vi "Initialize Tag.vi"(6 "Units":string, 8 "error in (no error)":errorcluster, 9 "Data Type":string(combo), 10 "Tag Path":string, 11 "Logger in.lvclass":refnum<class "Logger.lvclass">) -> (0 "error out":errorcluster, 3 "Logger out.lvclass":refnum<class "Logger.lvclass">)   [LabVIEW 2016, in "Logger.lvclass"]
uses:
  Logger.lvclass
  Logger.lvclass/Logger.ctl
  <vilib>/TagLibrary/Create Tag (String).vi
  <vilib>/TagLibrary/Create Tag (Int).vi
  <vilib>/TagLibrary/Create Tag (Double).vi
  <vilib>/TagLibrary/TagLibrary.lvlib
  <resource>/objmgr/niTag.rc
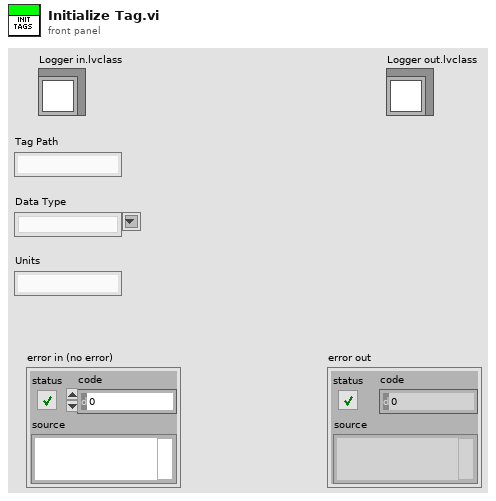
[diagram p1: front panel]
types:
  T1 = cluster{"Tag Reference":refnum<k21>, "Tag Units":string, "Tag Path":string, "Waveform":waveform(dbl), "Log":bool}
  T2 = cluster{"Tag Reference":refnum<k21>, "Tag Units":string, "Tag Path":string, "Waveform":waveform(dbl), "Log":bool}[]
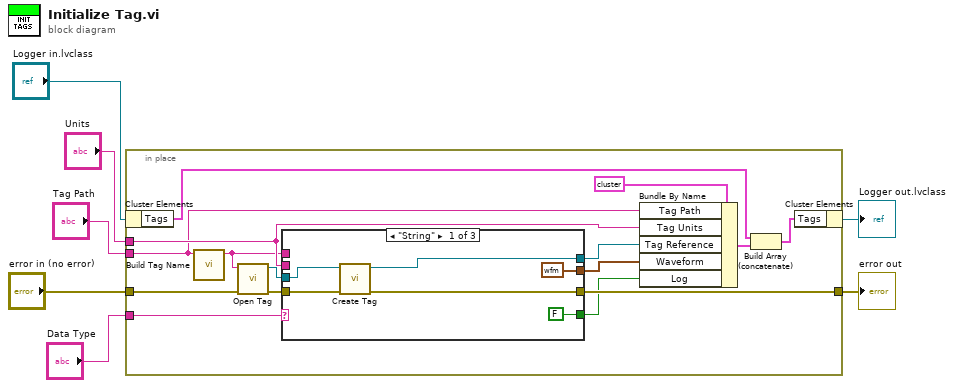
[diagram p0: block diagram]
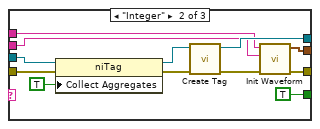
[diagram p2: hidden frame]
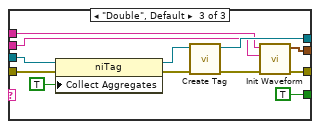
[diagram p3: hidden frame]
diagram:
  n1 = in-place {
    in-place-border: [w20] -> w7
    in-place-border: "Tag Path" -> [w8]
    in-place-border: "Data Type" -> [w19]
    in-place-border: "Units" -> [w16]
    in-place-border: "error in (no error)" -> [w15]
    n2 = in-place-cluster #1("Logger in.lvclass") -> ("Tags"=w11:T2)
    n3 = call "Build Tag Name.vi"("Tag"=w8) -> ("System Tag"=w12:string)  [unwired: 9 in, 1 out]
    n4 = call <vilib>:"Open Tag.vi"("error in (no error)"=w15, "tag path"=w12) -> ("error out"=w21:errorcluster, "tag reference out"=w22:refnum<k21>)  [unwired: 8 in]
    n5 = case shown="\"String\"" w19 {
      tunnel: w22 -> [w28 w40 w52]
      tunnel: w21 -> [w27 w37 w49]
      tunnel: [w25 w32 w44] -> w20
      tunnel: [w26 w35 w47] -> w17
      tunnel: [FALSE TRUE TRUE] -> w13
      tunnel: w16 -> [_ w29 w41]
      tunnel: [waveform(dbl) {"t0"=timestamp(0 s since 1904-01-01), "dt"=1.0, "Y"=[]} ("waveform") w31 w43] -> w14
      tunnel: w12 -> [_ w30 w42]
      frame "String" {
        n6 = call-poly <vilib>:"Create Tag.vi"("error in (no error)"=w27, "tag reference in"=w28) -> ("error out"=w25:errorcluster, "tag reference out"=w26:refnum<k21>)  [unwired: 8 in]
      }
      frame "Integer" {
        n7 = property class="niTag"(reference=w40, error in=w37, "Collect Aggregates"=TRUE) -> (reference out=w39:refnum<k21>, error out=w38:errorcluster)
        n8 = call-poly <vilib>:"Create Tag.vi"("error in (no error)"=w38, "tag reference in"=w39) -> ("error out"=w33:errorcluster, "tag reference out"=w35:refnum<k21>)  [unwired: 8 in]
        n9 = call "Init Waveform.vi"("error in (no error)"=w33, "Units"=w29, "System Tag"=w30) -> ("error out"=w32:errorcluster, "waveform"=w31:waveform(dbl))  [unwired: 7 in]
      }
      frame "Double", Default {
        n10 = property class="niTag"(reference=w52, error in=w49, "Collect Aggregates"=TRUE) -> (reference out=w51:refnum<k21>, error out=w50:errorcluster)
        n11 = call-poly <vilib>:"Create Tag.vi"("error in (no error)"=w50, "tag reference in"=w51) -> ("error out"=w45:errorcluster, "tag reference out"=w47:refnum<k21>)  [unwired: 8 in]
        n12 = call "Init Waveform.vi"("error in (no error)"=w45, "Units"=w41, "System Tag"=w42) -> ("error out"=w44:errorcluster, "waveform"=w43:waveform(dbl))  [unwired: 7 in]
      }
    }
    n13 = Bundle By Name(cluster=T1 {"Tag Reference"="", "Tag Units"="", "Tag Path"="", "Waveform"={"t0"=timestamp(0 s since 1904-01-01), "dt"=1.0, "Y"=[]}, "Log"=FALSE} ("Tag"), "Tag Path"=w8, "Tag Units"=w16, "Tag Reference"=w17, "Waveform"=w14, "Log"=w13) -> (w9:T1)
    n14 = Build Array (concatenate)(w11, w9) -> (w10:T2)
    n15 = in-place-cluster #1("Tags"=w10) -> (→"Logger out.lvclass":refnum<class "Logger.lvclass">)
  }
  "error out" <- w7
